vi "getMonth.vi"(8 "error in (no error)":errorcluster, 11 "WhichMonth in":refnum<class "WhichMonth.lvclass">) -> (0 "error out":errorcluster, 2 "Month":T1, 3 "WhichMonth out":refnum<class "WhichMonth.lvclass">)   [LabVIEW 2018, in "WhichMonth.lvclass"]
uses:
  WhichMonth.lvclass
  database/Month.ctl
  WhichMonth.lvclass/WhichMonth.ctl
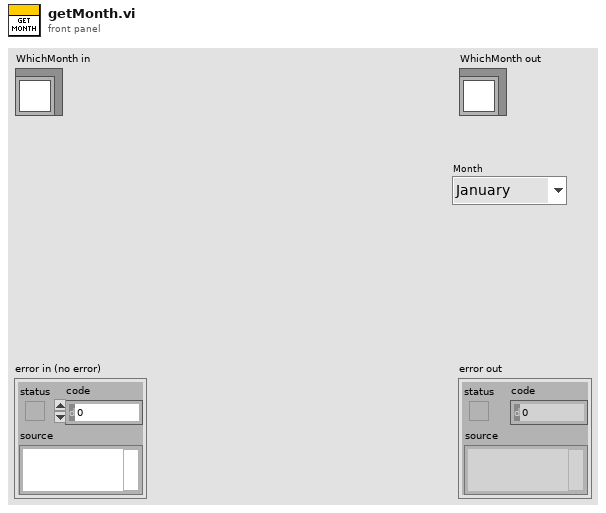
[diagram p1: front panel]
types:
  T1 = typedef "WhichMonth.lvclass/Month.ctl" = enum16{"January", "February", "March", "April", "May", "June", "July", "August", "September", "October", "November", "December"}
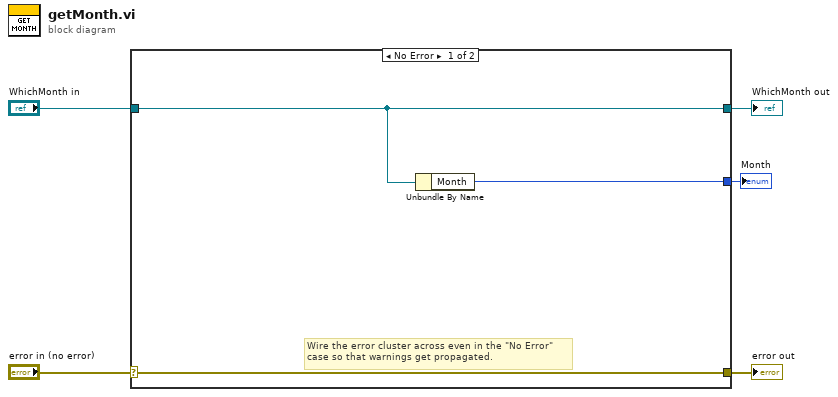
[diagram p0: block diagram]
diagram:
  n1 = case shown="No Error" "error in (no error)" {
    selector: "error in (no error)" -> [w8 w10]
    tunnel: [w8 w10] -> w4
    tunnel: [w7 w9] -> w2
    tunnel: "WhichMonth in" -> [w7 w9]
    tunnel: [w6 _] -> w1
    frame No Error {
      # "Wire the error cluster across even in the \"No Error\"\ncase so that warnings get propagated."
      n2 = Unbundle By Name(w7) -> ("Month"=w6:T1)
    }
    frame Error {
    }
  }
  "error out" <- w4
  "WhichMonth out" <- w2
  "Month" <- w1
